vi "NIIE_AssessRectangle.vi"(7 "Tool":T1, 10 "Coords":T3, 11 "Coords":T3) -> (3 "Rectangle Out":T2)   [LabVIEW 2021]
uses:
  <vilib>/Utility/miscctls.llb/LVPoint32TypeDef.ctl
  MB CORE/TypeDefs/Cluster_Button Draw Tools.ctl
  MB CORE/TypeDefs/Bool_Draw Tool.ctl
  MB CORE/TypeDefs/Bool_Line Tool.ctl
  MB CORE/TypeDefs/Bool_ColorExtractor Tool.ctl
  MB CORE/TypeDefs/Bool_Fill Tool.ctl
  MB CORE/TypeDefs/Bool_IERect Tool.ctl
  MB CORE/TypeDefs/Bool_FRect Tool.ctl
  MB CORE/TypeDefs/Bool_Circle Tool.ctl
  MB CORE/TypeDefs/Bool_FillCircle Tool.ctl
  MB CORE/TypeDefs/Bool_Eraser Tool.ctl
  MB CORE/TypeDefs/Bool_Text Tool.ctl
  MB CORE/TypeDefs/Bool_Selection Tool.ctl
  MB CORE/TypeDefs/Bool_Move Tool.ctl
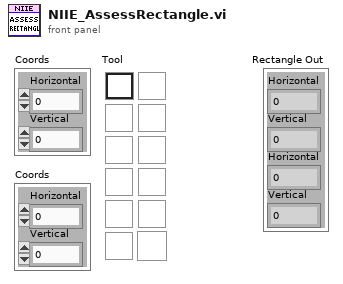
[diagram p1: front panel]
types:
  T1 = typedef "Cluster_Button Draw Tools.ctl" = enum32{"Pencil", "Line", "Dropper", "Fill", "Rectangle", "Filled Rectangle", "Ellipse", "Filled Ellipse", "Eraser", "Text", "Select", "Move"}
  T2 = cluster{"Horizontal":i32, "Vertical":i32, "Horizontal":i32, "Vertical":i32}
  T3 = typedef "LVPoint32TypeDef.ctl" = cluster{"Horizontal":i32, "Vertical":i32}
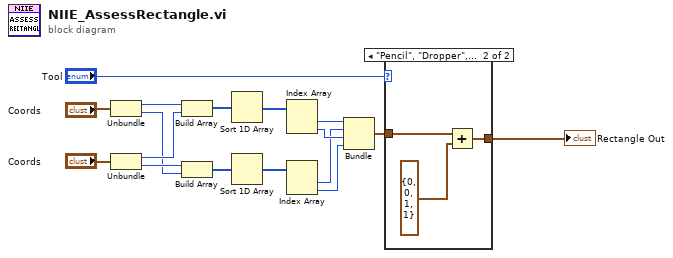
[diagram p0: block diagram]
diagram:
  n1 = Unbundle("Coords") -> ("Horizontal"=w15:i32, "Vertical"=w12:i32)
  n2 = Unbundle("Coords") -> ("Horizontal"=w14:i32, "Vertical"=w13:i32)
  n3 = Build Array(w15, w14) -> (w11:i32[])
  n4 = Build Array(w13, w12) -> (w10:i32[])
  n5 = Sort 1D Array(array=w11) -> (sorted array=w9:i32[])
  n6 = Sort 1D Array(array=w10) -> (sorted array=w8:i32[])
  n7 = Index Array(array=w9) -> (element #1=w7:i32, element #2=w6:i32)  [unwired: 2 in]
  n8 = Index Array(array=w8) -> (element #1=w5:i32, element #2=w4:i32)  [unwired: 2 in]
  n9 = Bundle("Horizontal"=w7, "Vertical"=w5, "Horizontal"=w6, "Vertical"=w4) -> (w2:T2)  [unwired: 1 out]
  n10 = case shown="\"Pencil\", \"Dropper\", \"Rectangle\", \"Eraser\"" "Tool" {
    tunnel: w2 -> [w18 w21]
    tunnel: [w18 w19] -> w1
    frame Default {
    }
    frame "Pencil", "Dropper", "Rectangle", "Eraser" {
      n11 = Add(x=w21, y=T2 {"Horizontal"=0, "Vertical"=0, "Horizontal"=1, "Vertical"=1} ("output cluster")) -> (x+y=w19:T2)
    }
  }
  "Rectangle Out" <- w1
